vi "Create Message Queues Facilitating Data Acquisition and Logging.vi"(8 "error in (no error)":errorcluster caption="错误输入（无错误）") -> (0 "error out":errorcluster caption="错误输出")   [LabVIEW 2013, in "Message Queue.lvlib"]
doc: "本VI用于创建应用程序所需的所有消息队列。如应用程序需要两个以上消息队列，可右键单击上面的“消息队列”常量并选择“打开自定义类型”，将新的消息队列添加至该自定义类型，然后通过本VI进行初始化。"
uses:
  Message Queue.lvlib
panel:
  out "Queues for Data Acquistion, Logging and Transmission":T1 caption="数据采集、记录与传输中应用的队列"
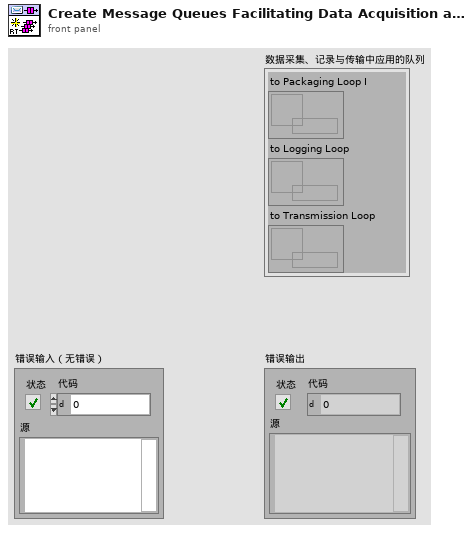
[diagram p1: front panel]
types:
  T1 = cluster{"to Packaging Loop I":refnum<queue>, "to Logging Loop":refnum<queue>, "to Transmission Loop":refnum<queue>}
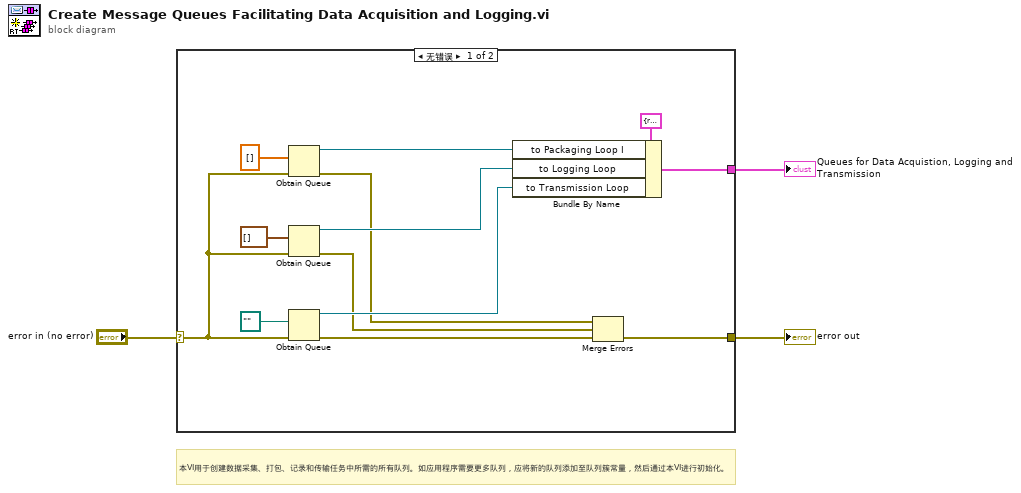
[diagram p0: block diagram]
diagram:
  # "本VI用于创建数据采集、打包、记录和传输任务中所需的所有队列。如应用程序需要更多队列，应将新的队列添加至队列簇常量，然后通过本VI进行初始化。"
  n1 = case shown="无错误" "error in (no error)" {
    selector: "error in (no error)" -> [w9 w17]
    tunnel: [w11 w17] -> w3
    tunnel: [w14 _] -> w1
    frame No Error {
      n2 = Obtain Queue(element data type=dbl[] [], error in (no error)=w9) -> (queue out=w12:refnum<queue>, error out=w13:errorcluster)  [unwired: 3 in, 1 out]
      n3 = Obtain Queue(element data type=waveform(dbl)[] [], error in (no error)=w9) -> (queue out=w15:refnum<queue>, error out=w8:errorcluster)  [unwired: 3 in, 1 out]
      n4 = Obtain Queue(element data type=path "", error in (no error)=w9) -> (queue out=w16:refnum<queue>, error out=w10:errorcluster)  [unwired: 3 in, 1 out]
      n5 = Bundle By Name(cluster=T1 {"to Packaging Loop I"=refnum, "to Logging Loop"=refnum, "to Transmission Loop"=refnum}, "to Packaging Loop I"=w12, "to Logging Loop"=w15, "to Transmission Loop"=w16) -> (w14:T1)
      n6 = Merge Errors(w13, w8, w10) -> (w11:errorcluster)
    }
    frame Error {
    }
  }
  "error out" <- w3
  "Queues for Data Acquistion, Logging and Transmission" <- w1
